vi "Allgemein_Length_By_KeyIndex.vi"(6 "Teil-Array":string[](array[string]), 11 "Key Index Array (Eingang)":i32[](array[numeric])) -> (2 "Sorted Length Array":i32[](array[numeric]), 3 "Length Array  (Ausgang)":i32[](array[numeric]), 5 "Sorted Array":i32[](array[numeric]), 7 "Index Array":i32[](array[numeric]))   [LabVIEW 2020, in "System Einstellungen V2.lvlib"]
doc: "Bestimmen der Länge der Einträge in Dateien mit Schlüssel (Key) wie [Optionen] [Gasteiler].\nEingang: Array mit Indizex der Keys im Text.\nAusgang: Länge der jeweiligen Blöcke, ess muss noch -1 abgezogen werden.\nBeim letzten Eintrag wird als Länge die Länge von Key bis zum Ende oder bis zur nächsten \"[\" angegeben.\nIst kein Eintrag vorhanden (-1 im Eingang), wird 0 zurück gegeben, das muss extern berücksichtigt werden.\nRIW, 2022-12-13"
uses:
  System Einstellungen V2.lvlib
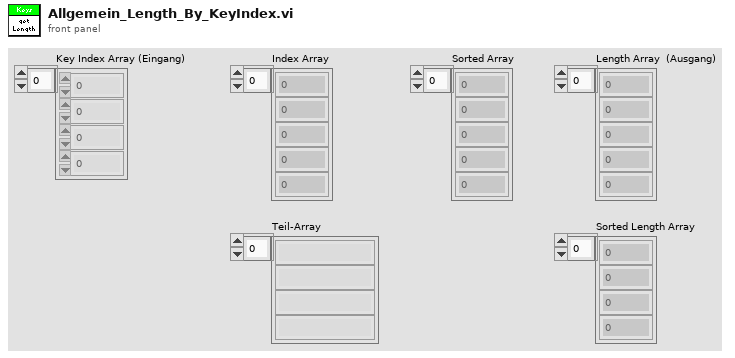
[diagram p1: front panel]
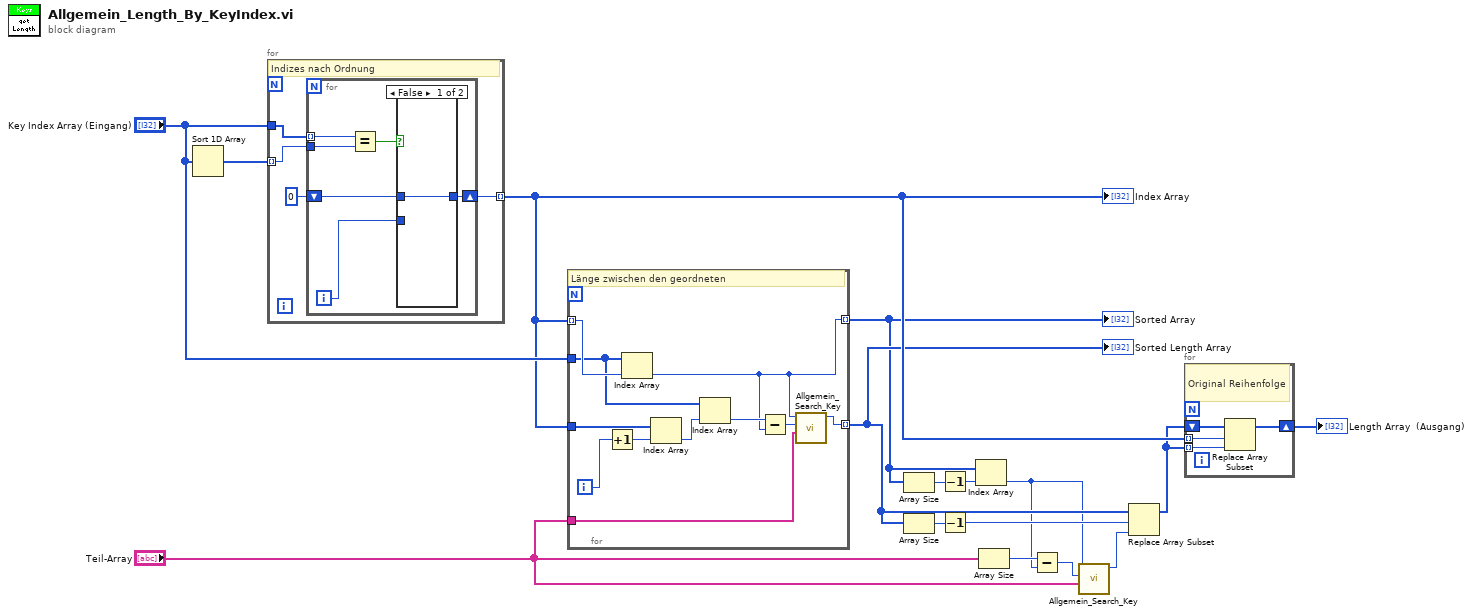
[diagram p0: block diagram]
diagram:
  n1 = Sort 1D Array(array="Key Index Array (Eingang)") -> (sorted array=w3:i32[])
  n2 = for {
    tunnel: "Key Index Array (Eingang)" -> [w20]
    tunnel: w3 -> [w19] mode=indexing
    tunnel: [w18] -> w15 mode=indexing
    # "Indizes nach Ordnung"
    n3 = for {
      tunnel: w20 -> [w26] mode=indexing
      tunnel: w19 -> [w25]
      shift-right: [w23] -> w18
      shift-left: 0 -> [w22]
      i -> [w21]
      n4 = Equal?(x=w26, y=w25) -> (x = y?=w24:bool)
      n5 = case shown="False" w24 {
        tunnel: w21 -> [_ w28]
        tunnel: [w27 w28] -> w23
        tunnel: w22 -> [w27 _]
        frame False {
        }
        frame True {
        }
      }
    }
  }
  "Index Array" <- w15
  n6 = for {
    tunnel: w15 -> [w39] mode=indexing
    tunnel: "Key Index Array (Eingang)" -> [w35]
    tunnel: w15 -> [w38]
    tunnel: [w30] -> w13 mode=indexing
    tunnel: [w32] -> w11 mode=indexing
    tunnel: "Teil-Array" -> [w29]
    i -> [w37]
    # "Länge zwischen den geordneten"
    n7 = Increment(x=w37) -> (x+1=w36:i32)
    n8 = Index Array(array=w35, index=w39) -> (element=w32:i32)
    n9 = Index Array(array=w38, index=w36) -> (element=w34:i32)
    n10 = Index Array(array=w35, index=w34) -> (element=w33:i32)
    n11 = Subtract(x=w33, y=w32) -> (x-y=w31:i32)
    n12 = call "Allgemein_Search_Key.vi"("Teil-Array"=w29, "length (Eingang)"=w31, "index of Options"=w32) -> ("length (Ausgang)"=w30:i32)  [unwired: 8 in]
  }
  "Sorted Length Array" <- w13
  "Sorted Array" <- w11
  n13 = Array Size(array=w11) -> (size(s)=w10:i32)
  n14 = Array Size(array=w13) -> (size(s)=w14:i32)
  n15 = Decrement(x=w10) -> (x-1=w9:i32)
  n16 = Decrement(x=w14) -> (x-1=w12:i32)
  n17 = Index Array(array=w11, index=w9) -> (element=w7:i32)
  n18 = Array Size(array="Teil-Array") -> (size(s)=w8:i32)
  n19 = Subtract(x=w8, y=w7) -> (x-y=w6:i32)
  n20 = call "Allgemein_Search_Key.vi"("Teil-Array"="Teil-Array", "length (Eingang)"=w6, "index of Options"=w7) -> ("length (Ausgang)"=w5:i32)  [unwired: 8 in]
  n21 = Replace Array Subset(array=w13, new element=w5, index=w12) -> (w2:i32[])
  n22 = for {
    tunnel: w15 -> [w43] mode=indexing
    tunnel: w2 -> [w42] mode=indexing
    shift-right: [w41] -> w1
    shift-left: w2 -> [w40]
    # "Original Reihenfolge"
    n23 = Replace Array Subset(array=w40, new element=w42, index=w43) -> (w41:i32[])
  }
  "Length Array  (Ausgang)" <- w1
